vi "Init.vi"(8 "error in (no error)":errorcluster, 11 "Mock In":refnum<class "Mock.lvclass">) -> (0 "error out":errorcluster, 3 "Mock Out":refnum<class "Mock.lvclass">)   [LabVIEW 2020, in "Mock.lvclass"]
uses:
  Mock.lvclass
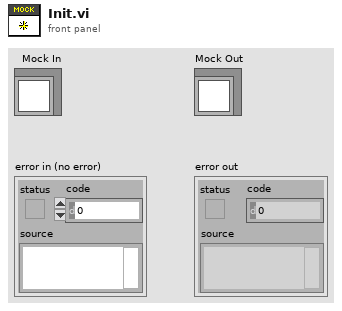
[diagram p1: front panel]
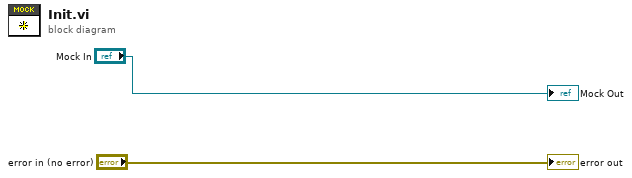
[diagram p0: block diagram]
diagram:
  "error out" <- "error in (no error)"
  "Mock Out" <- "Mock In"
